vi "Import User Defined Messages.vi"(8 "error in (no error)":errorcluster, 11 "Node Ptr":u64 format="%.0x") -> (0 "error out":errorcluster)   [LabVIEW 2019, in "Diagnostics Addon System Explorer.lvlib"]
uses:
  Diagnostics Addon System Explorer.lvlib
  Types/UserDefinedMessage.Export.ctl
  Types/CmdResp.Export.ctl
  Addon Shared/Types/Signal.ctl
  Addon Shared/Types/Type.ctl
  Addon Shared/Diagnostics Addon Shared.lvlib
  <vilib>/NI VeriStand/Custom Device Tools/Custom Device Utility Library/Custom Device Utility Library.lvlib
  <vilib>/NI VeriStand/Custom Device API/Custom Device API.lvlib
panel:
  in  "Tag":string
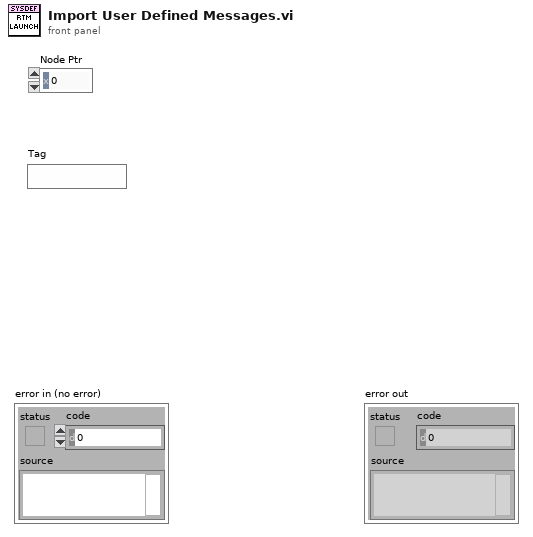
[diagram p1: front panel]
types:
  T1 = typedef "Diagnostics Addon System Explorer.lvlib/UserDefinedMessage.Export.ctl" = cluster{"Name":string, "Signals":T2}
  T2 = typedef "Diagnostics Addon System Explorer.lvlib/CmdResp.Export.ctl" = cluster{"Cmd":T3[], "Response":T3[]}
  T3 = typedef "Diagnostics Addon Shared.lvlib/Signal.ctl" = cluster{"Start Bit":u32, "Length":u32, "Scaling Factor":dbl, "Scaling Offset":dbl, "Minimum":dbl, "Maximum":dbl, "Data Type":u32, "Byte Order":u32, "Default Value":dbl, "Name":string, "Units":string}
  T4 = typedef "Diagnostics Addon Shared.lvlib/Type.ctl" = enum16{"DID", "CDID", "PID", "CPID", "Read Memory", "Write Memory", "IO Control", "Routine Start", "Routine Request", "Routine Stop", "User Defined", "DTC Control", "Clear DTCs", "Read DTCs", "Start DTCs", "DTC Change Count", "Tester Present", "Unlock ECU", "Reset ECU", "Diag Session Control", "Communication Control", "DPID Control", "Poll Control", "Diag CAN Control"}
  T5 = typedef "Custom Device API.lvlib/Custom Device Item Ref.ctl" = u64
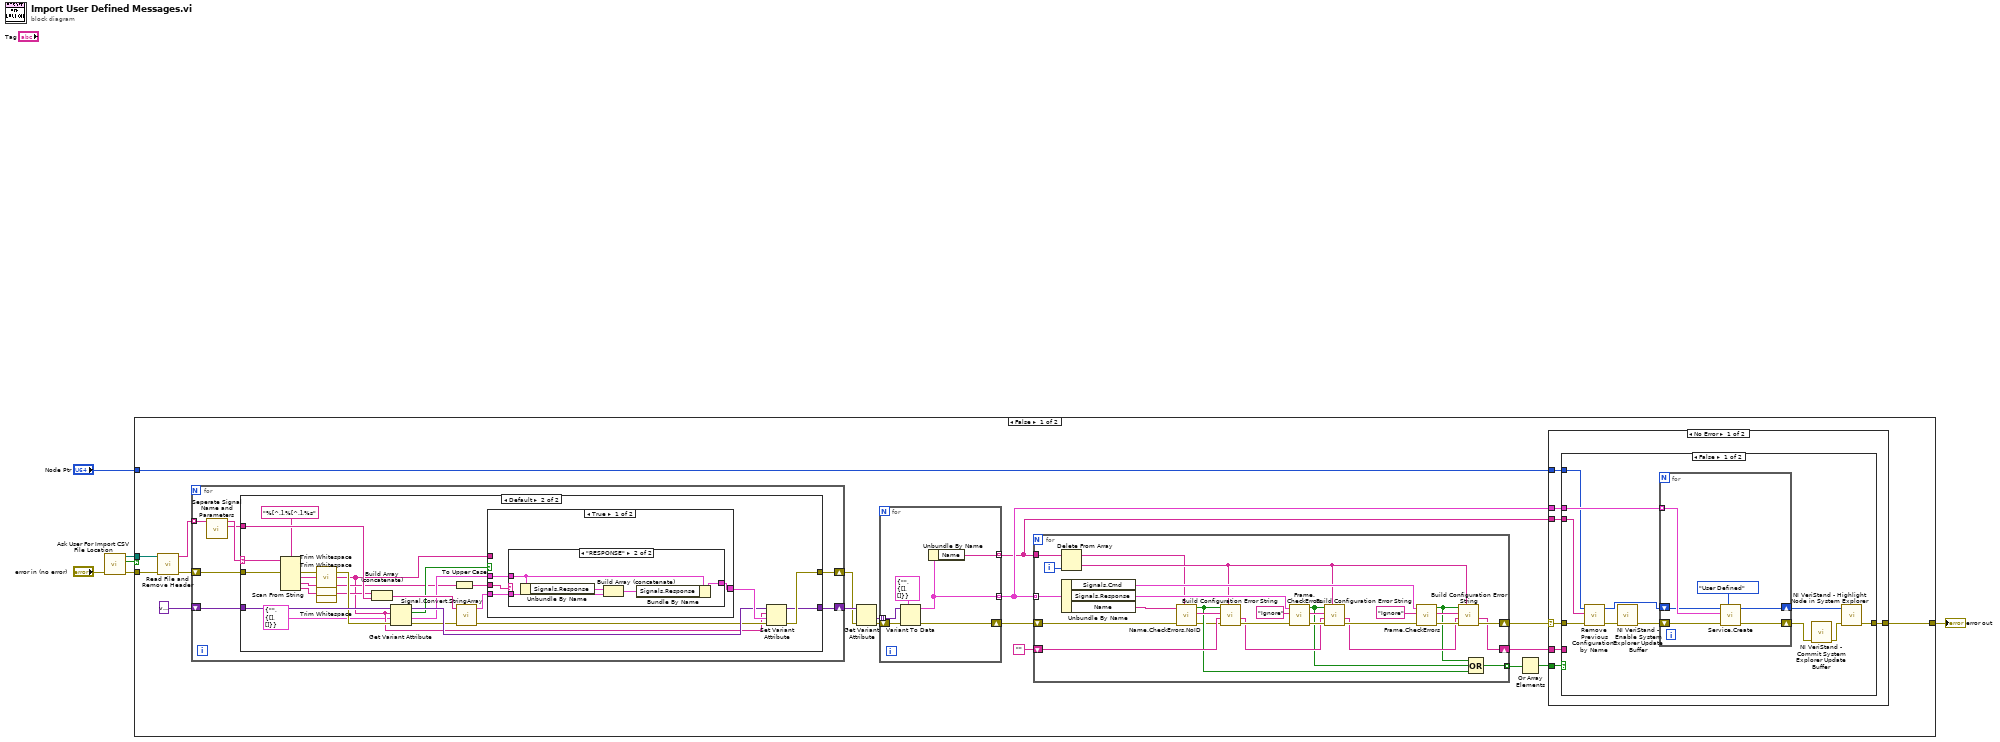
[diagram p0: block diagram]
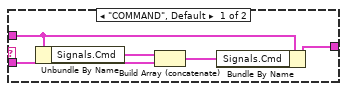
[diagram p3: hidden frame]
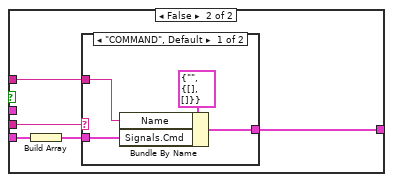
[diagram p4: hidden frame]
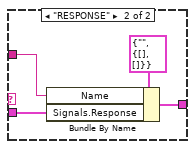
[diagram p5: hidden frame]
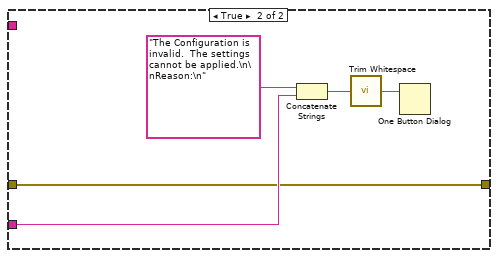
[diagram p6: hidden frame]
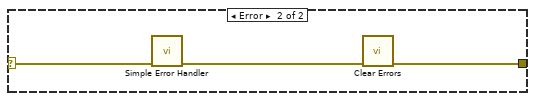
[diagram p7: hidden frame]
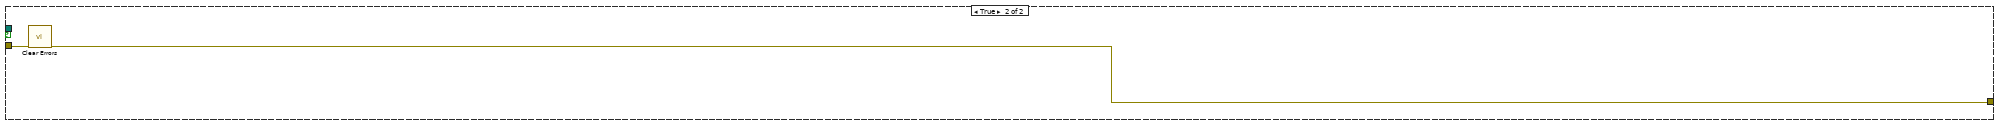
[diagram p8: hidden frame]
diagram:
  n1 = call "Ask User For Import CSV File Location.vi"("error in (no error)"="error in (no error)") -> ("error out"=w2:errorcluster, "cancelled"=w3:bool, "selected path"=w1:path)  [unwired: 8 in]
  n2 = case shown="False" w3 {
    tunnel: w2 -> [w25 w153]
    tunnel: w1 -> [w24 _]
    tunnel: "Node Ptr" -> [w10 _]
    tunnel: [w12 w152] -> w5
    frame False {
      n3 = call "Read File and Remove Header.vi"("error in (no error)"=w25, "selected path"=w24) -> ("error out"=w23:errorcluster, "Array"=w8:string[])  [unwired: 8 in]
      n4 = for {
        tunnel: w8 -> [w32] mode=indexing
        shift-right: [w29] -> w20
        shift-left: w23 -> [w30]
        shift-right: [w28] -> w21
        shift-left: variant -> [w31]
        n5 = call "Seperate Signal Name and Parameters.vi"("String"=w32) -> ("Signal Parameters"=w26:string[], "Signal Name"=w27:string)  [unwired: 9 in]
        n6 = case shown="Default" w27 {
          selector: w27 -> [_ w44]
          tunnel: w26 -> [_ w58]
          tunnel: w31 -> [w34 w55]
          tunnel: w30 -> [w33 w54]
          tunnel: [w33 w50] -> w29
          tunnel: [w34 w49] -> w28
          frame "" {
          }
          frame Default {
            n7 = Scan From String(format string="%[^.].%[^.].%s", input string=w44, error in=w54) -> (error out=w48:errorcluster, output 1=w39:string, output 2=w38:string, output 3=w37:string)  [unwired: 4 in, 2 out]
            n8 = call <vilib>:"Trim Whitespace.vi"("string"=w39) -> ("trimmed string"=w36:string)  [unwired: 1 in]
            n9 = call <vilib>:"Trim Whitespace.vi"("string"=w38) -> ("trimmed string"=w41:string)  [unwired: 1 in]
            n10 = call <vilib>:"Trim Whitespace.vi"("string"=w37) -> ("trimmed string"=w40:string)  [unwired: 1 in]
            n11 = Build Array (concatenate)(w40, w58) -> (w56:string[])
            n12 = Get Variant Attribute(Variant=w55, name=w36, default value (empty Variant)=T1 {"Name"="", "Signals"={"Cmd"=[], "Response"=[]}} ("IO Control"), error in=w48) -> (duplicate Variant=w52:variant, found=w46:bool, value=w45:T1, error out=w47:errorcluster)
            n13 = To Upper Case(1:w41) -> (0:w43:string)
            n14 = call "Signal.Convert.StringArray.vi"("error in (no error)"=w47, "Signal Parameters"=w56) -> ("error out"=w51:errorcluster, "Signal Parameters"=w57:T3)  [unwired: 8 in]
            n15 = case shown="True" w46 {
              tunnel: w57 -> [w61 w77]
              tunnel: w36 -> [_ w76]
              tunnel: [w60 w74] -> w53
              tunnel: w45 -> [w62 _]
              tunnel: w43 -> [w59 w73]
              frame True {
                n16 = case shown="\"RESPONSE\"" w59 {
                  tunnel: w62 -> [w67 w72]
                  tunnel: w61 -> [w65 w70]
                  tunnel: [w63 w68] -> w60
                  frame "COMMAND", Default {
                    n17 = Unbundle By Name(w67) -> ("Signals.Cmd"=w66:T3[])
                    n18 = Build Array (concatenate)(w66, w65) -> (w64:T3[])
                    n19 = Bundle By Name(cluster=w67, "Signals.Cmd"=w64) -> (w63:T1)
                  }
                  frame "RESPONSE" {
                    n20 = Unbundle By Name(w72) -> ("Signals.Response"=w71:T3[])
                    n21 = Build Array (concatenate)(w71, w70) -> (w69:T3[])
                    n22 = Bundle By Name(cluster=w72, "Signals.Response"=w69) -> (w68:T1)
                  }
                }
              }
              frame False {
                n23 = Build Array(w77) -> (w75:T3[])
                n24 = case shown="\"COMMAND\", Default" w73 {
                  tunnel: w76 -> [w81 w85]
                  tunnel: w75 -> [w80 w84]
                  tunnel: [w79 w83] -> w74
                  frame "COMMAND", Default {
                    n25 = Bundle By Name(cluster=T1 {"Name"="", "Signals"={"Cmd"=[], "Response"=[]}} ("IO Control"), "Name"=w81, "Signals.Cmd"=w80) -> (w79:T1)
                  }
                  frame "RESPONSE" {
                    n26 = Bundle By Name(cluster=T1 {"Name"="", "Signals"={"Cmd"=[], "Response"=[]}} ("IO Control"), "Name"=w85, "Signals.Response"=w84) -> (w83:T1)
                  }
                }
              }
            }
            n27 = Set Variant Attribute(Variant=w52, name=w36, value=w53, error in=w51) -> (Variant out=w49:variant, error out=w50:errorcluster)  [unwired: 1 out]
          }
        }
      }
      n28 = Get Variant Attribute(Variant=w21, error in=w20) -> (values=w19:variant[], error out=w18:errorcluster)  [unwired: 2 in, 2 out]
      n29 = for {
        tunnel: w19 -> [w91] mode=indexing
        shift-right: [w89] -> w11
        shift-left: w18 -> [w90]
        tunnel: [w88] -> w13 mode=indexing
        tunnel: [w86] -> w7 mode=indexing
        n30 = Variant To Data(error in=w90, type=T1 {"Name"="", "Signals"={"Cmd"=[], "Response"=[]}} ("IO Control"), Variant=w91) -> (data=w88:T1, error out=w89:errorcluster)
        n31 = Unbundle By Name(w88) -> ("Name"=w86:string)
      }
      n32 = for {
        tunnel: w13 -> [w119] mode=indexing
        shift-right: [w118] -> w9
        shift-left: w11 -> [w92]
        shift-right: [w103] -> w14
        shift-left: "" -> [w106]
        tunnel: [w101] -> w16 mode=indexing
        tunnel: w7 -> [w117]
        i -> [w116]
        n33 = Delete From Array(array=w117, index=w116) -> (deleted portion=w99:string, array with subset deleted=w97:string[])  [unwired: 1 in]
        n34 = Unbundle By Name(w119) -> ("Signals.Cmd"=w113:T3[], "Signals.Response"=w115:T3[], "Name"=w96:string)
        n35 = call "Name.CheckErrors.NoID.vi"("Existing Frames"=w97, "error in (no error)"=w92, "Name"=w96) -> ("error out"=w93:errorcluster, "Error String"=w95:string, "Error?"=w94:bool)  [unwired: 6 in]
        n36 = call "Build Configuration Error String.vi"("Name"=w99, "error in (no error)"=w93, "String in"=w106, "Error"=w95, "Error?"=w94) -> ("error out"=w111:errorcluster, "String out"=w105:string)  [unwired: 5 in]
        n37 = call "Frame.CheckErrors.vi"("error in (no error)"=w111, "Name"="Ignore", "Signals"=w115) -> ("error out"=w110:errorcluster, "Error Type"=w109:string, "Error?"=w102:bool)  [unwired: 6 in]
        n38 = call "Build Configuration Error String.vi"("Name"=w99, "error in (no error)"=w110, "String in"=w105, "Error"=w109, "Error?"=w102) -> ("error out"=w108:errorcluster, "String out"=w104:string)  [unwired: 5 in]
        n39 = call "Frame.CheckErrors.vi"("error in (no error)"=w108, "Name"="Ignore", "Signals"=w113) -> ("error out"=w114:errorcluster, "Error Type"=w107:string, "Error?"=w98:bool)  [unwired: 6 in]
        n40 = call "Build Configuration Error String.vi"("Name"=w99, "error in (no error)"=w114, "String in"=w104, "Error"=w107, "Error?"=w98) -> ("error out"=w118:errorcluster, "String out"=w103:string)  [unwired: 5 in]
        n41 = Compound Arithmetic op=OR(w98, w102, w94) -> (w101:bool)
      }
      n42 = Or Array Elements(Boolean array=w16) -> (logical OR=w15:bool)
      n43 = case shown="No Error" w9 {
        selector: w9 -> [w122 w151]
        tunnel: w15 -> [w126 _]
        tunnel: w14 -> [w125 _]
        tunnel: w13 -> [w124 _]
        tunnel: [w123 w149] -> w12
        tunnel: w10 -> [w121 _]
        tunnel: w7 -> [w120 _]
        frame No Error {
          n44 = case shown="False" w126 {
            tunnel: w125 -> [_ w146]
            tunnel: w122 -> [w131 w145]
            tunnel: w124 -> [w133 _]
            tunnel: [w132 w145] -> w123
            tunnel: w121 -> [w130 _]
            tunnel: w120 -> [w127 _]
            frame False {
              n45 = call "Remove Previous Configurations by Name.vi"("error in (no error)"=w131, "Imported Names"=w127, "Node In"=w130) -> ("error out"=w129:errorcluster, "Node Out"=w128:T5)  [unwired: 7 in]
              n46 = call <vilib>:"NI VeriStand - Enable System Explorer Update Buffer.vi"("error in (no error)"=w129) -> ("error out"=w136:errorcluster)  [unwired: 10 in]
              n47 = for {
                shift-right: [w140] -> w135
                shift-left: w136 -> [w139]
                shift-right: [w141] -> w137
                shift-left: w128 -> [w142]
                tunnel: w133 -> [w143] mode=indexing
                n48 = call "Service.Create.vi"("Type"=Type."User Defined", "error in (no error)"=w139, "Variant"=w143, "Section Ptr"=w142) -> ("error out"=w140:errorcluster, "Parent Ref out"=w141:T5)  [unwired: 6 in]
              }
              n49 = call <vilib>:"NI VeriStand - Commit System Explorer Update Buffer.vi"("error in (no error)"=w135) -> ("error out"=w134:errorcluster)  [unwired: 10 in]
              n50 = call <vilib>:"NI VeriStand - Highlight Node in System Explorer.vi"("error in (no error)"=w134, "Item Ref in"=w137) -> ("error out"=w132:errorcluster)  [unwired: 8 in, 1 out]
            }
            frame True {
              n51 = Concatenate Strings("The Configuration is invalid.  The settings cannot be applied.\n\nReason:\n" ("message"), w146) -> (w148:string)
              n52 = call <vilib>:"Trim Whitespace.vi"("string"=w148) -> ("trimmed string"=w144:string)  [unwired: 1 in]
              n53 = One Button Dialog(message=w144) -> ()  [unwired: 1 in, 1 out]
            }
          }
        }
        frame Error {
          n54 = call <vilib>:"Simple Error Handler.vi"("error in (no error)"=w151) -> ("error out"=w150:errorcluster)  [unwired: 4 in, 4 out]
          n55 = call <vilib>:"Clear Errors.vi"("error in (no error)"=w150) -> ("error out"=w149:errorcluster)  [unwired: 5 in, 1 out]
        }
      }
    }
    frame True {
      n56 = call <vilib>:"Clear Errors.vi"("error in (no error)"=w153) -> ("error out"=w152:errorcluster)  [unwired: 5 in, 1 out]
    }
  }
  "error out" <- w5
